vi "WLAN - Test - UTIL - FormatResult(scalar).vi"(7 "Number":dbl) -> (8 "2nd order decimal":dbl format="%6.2f")   [LabVIEW 2011]
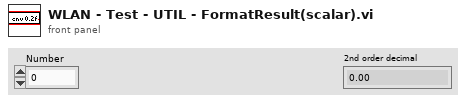
[diagram p1: front panel]
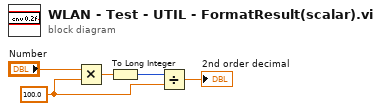
[diagram p0: block diagram]
diagram:
  w2 = 100.0 ("y")
  n1 = Multiply(x="Number", y=w2) -> (x*y=w4:dbl)
  n2 = To Long Integer(number=w4) -> (32bit integer=w3:i32)
  n3 = Divide(x=w3, y=w2) -> (x/y=→"2nd order decimal":dbl)
